vi "volume integrator 2016.vi"(4 "Previous Time (sec)":dbl, 6 "Flow":dbl format="%.2f", 7 "Total Volume in":dbl format="%.2f") -> (0 "Current Time (sec)":dbl, 3 "Total Volume Out":dbl format="%.2f")   [LabVIEW 2016]
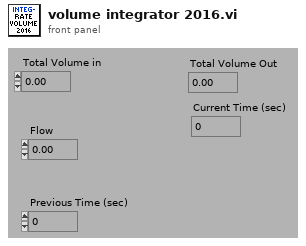
[diagram p1: front panel]
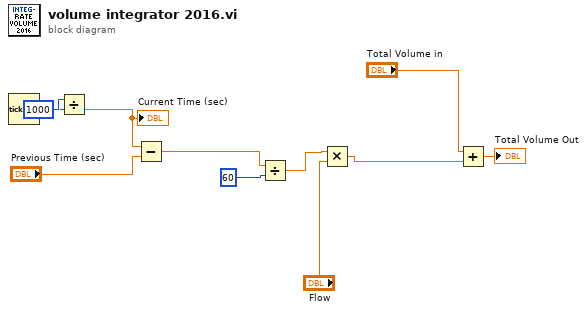
[diagram p0: block diagram]
diagram:
  n1 = Tick Count (ms)() -> (millisecond timer value=w5:u32)
  n2 = Divide(x=w5, y=u32 1000) -> (x/y=w6:dbl)
  "Current Time (sec)" <- w6
  n3 = Subtract(x=w6, y="Previous Time (sec)") -> (x-y=w3:dbl)
  n4 = Divide(x=w3, y=60) -> (x/y=w2:dbl)
  n5 = Multiply(x=w2, y="Flow") -> (x*y=w1:dbl)
  n6 = Add(x="Total Volume in", y=w1) -> (x+y=→"Total Volume Out":dbl)
